vi "Check for Gauge Alarm.vi"(2 "Knob Refnum":refnum<vi>) -> ()   [LabVIEW 2012]
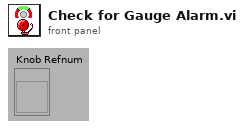
[diagram p1: front panel]
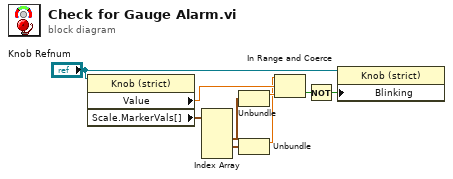
[diagram p0: block diagram]
diagram:
  n1 = property on="Property Node" class="Knob (strict)"(reference="Knob Refnum") -> ("Value"=w7:dbl, "Scale.MarkerVals[]"=w5:cluster{dbl, u32}[])  [unwired: 1 in, 2 out]
  n2 = Index Array(array=w5) -> (element #2=w4:cluster{dbl, u32}, element #3=w3:cluster{dbl, u32})  [unwired: 4 in, 2 out]
  n3 = Unbundle(w4) -> (w2:dbl)  [unwired: 1 out]
  n4 = Unbundle(w3) -> (w1:dbl)  [unwired: 1 out]
  n5 = In Range and Coerce(upper limit=w1, x=w7, lower limit=w2) -> (In Range?=w8:bool)  [unwired: 1 out]
  n6 = Not(x=w8) -> (.not. x?=w9:bool)
  n7 = property on="Property Node" class="Knob (strict)"(reference="Knob Refnum", "Blinking"=w9) -> ()  [unwired: 1 in, 2 out]
